vi "Remove WebSockets from palette.vi"() -> ()   [LabVIEW 2013]
uses:
  <vilib>/Palette API/Palette Menu/Public Type Define/Palette type.ctl
  <vilib>/Palette API/Palette Menu/Palette Menu.lvlib
panel:
  out "error out":errorcluster
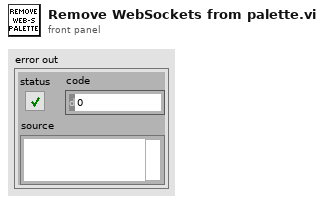
[diagram p1: front panel]
types:
  T1 = typedef "Palette Menu.lvlib/Palette type.ctl" = i32
  T2 = typedef "Palette Menu.lvlib/Palette Data.ctl" = cluster{"display name":string, "view format":T3, "palette width":i16, "items":T4, "256 color icon":picture, "B&W color icon":picture, "help information":T6, "palette description":string, "synchronize information":T7}
  T3 = typedef "Palette Menu.lvlib/View Format.ctl" = u16
  T4 = typedef "Palette Menu.lvlib/Items.ctl" = T5[]
  T5 = typedef "Palette Menu.lvlib/Item.ctl" = cluster{"item path":path, "library path (.lvlib)":path, "use default lvlib palette":bool, "short name":string, "place VI contents":bool, "hide synchronized item":bool, "reserve spot for synch item":bool, "configure when placing VI contents":bool}
  T6 = typedef "Palette Menu.lvlib/Help Info.ctl" = cluster{"help tag":string, "help file path ":path}
  T7 = typedef "Palette Menu.lvlib/Synchronize Info.ctl" = cluster{"synchronize with directory":bool, "synchronize directory path":path}
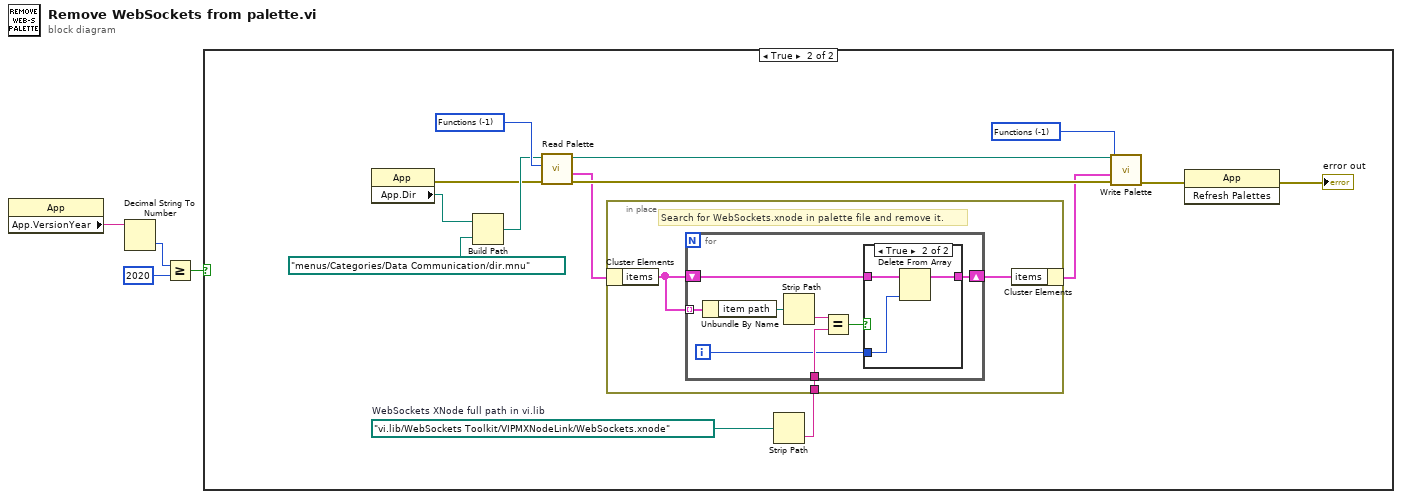
[diagram p0: block diagram]
diagram:
  n1 = property class="App"() -> ("App.VersionYear"=w2:string)  [unwired: 2 in, 2 out]
  n2 = Decimal String To Number(string=w2) -> (number=w4:i32)  [unwired: 2 in, 1 out]
  n3 = Greater Or Equal?(x=w4, y=2020) -> (x >= y?=w1:bool)
  n4 = case shown="True" w1 {
    frame False {
      # "No ops"
    }
    frame True {
      w10 = T1 -1 items=["Functions"=-1, "Controls"=-2] ("palette type")
      w14 = path "vi.lib/WebSockets Toolkit/VIPMXNodeLink/WebSockets.xnode"  # WebSockets XNode full path in vi.lib
      w18 = T1 -1 items=["Functions"=-1, "Controls"=-2] ("palette type")
      n5 = property class="App"() -> (error out=w9:errorcluster, "App.Dir"=w15:path)  [unwired: 2 in, 1 out]
      n6 = Build Path(base path=w15, name or relative path=path "menus/Categories/Data Communication/dir.mnu") -> (appended path=w16:path)
      n7 = call <vilib>:"Read Palette.vi"("error in (no error)"=w9, "palette type"=w18, "palette path"=w16) -> ("error out"=w8:errorcluster, "palette data"=w6:T2, "duplicate palette path"=w13:path)  [unwired: 1 in, 5 out]
      n8 = Strip Path(path=w14) -> (name=w7:string)  [unwired: 1 out]
      n9 = in-place {
        in-place-border: w7 -> [w21]
        # "Search for WebSockets.xnode in palette file and remove it."
        n10 = in-place-cluster #1(w6) -> ("items"=w20:T4)
        n11 = for {
          tunnel: w20 -> [w29] mode=indexing
          tunnel: w21 -> [w26]
          shift-right: [w22] -> w19
          shift-left: w20 -> [w24]
          i -> [w23]
          n12 = Unbundle By Name(w29) -> ("item path"=w28:path)
          n13 = Strip Path(path=w28) -> (name=w27:string)  [unwired: 1 out]
          n14 = Equal?(x=w27, y=w26) -> (x = y?=w25:bool)
          n15 = case shown="True" w25 {
            tunnel: w24 -> [w30 w32]
            tunnel: w23 -> [_ w33]
            tunnel: [w30 w31] -> w22
            frame False {
            }
            frame True {
              n16 = Delete From Array(array=w32, index=w33) -> (array with subset deleted=w31:T4)  [unwired: 1 in, 1 out]
            }
          }
        }
        n17 = in-place-cluster #1("items"=w19) -> (w5:T2)
      }
      n18 = call <vilib>:"Write Palette.vi"("error in (no error)"=w8, "palette data"=w5, "palette type"=w10, "palette path"=w13) -> ("error out"=w11:errorcluster)  [unwired: 1 in, 6 out]
      n19 = invoke class="App" method="Refresh Palettes"(error in=w11) -> (error out=→"error out":errorcluster)  [unwired: 2 in, 2 out]
    }
  }
